vi "Write Rotronic.vi"(8 "error in":errorcluster, 10 "Rotronic":cluster{"RH":sgl, "T":sgl}, 11 "tCRD Data in":refnum<class "tCRD Data.lvclass">) -> (0 "error out":errorcluster, 3 "tCRD Data out":refnum<class "tCRD Data.lvclass">)   [LabVIEW 2015, in "tCRD Data.lvclass"]
uses:
  tCRD Data.lvclass
  tCRD Data.lvclass/tCRD Data.ctl
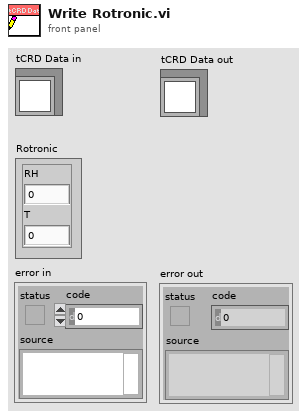
[diagram p1: front panel]
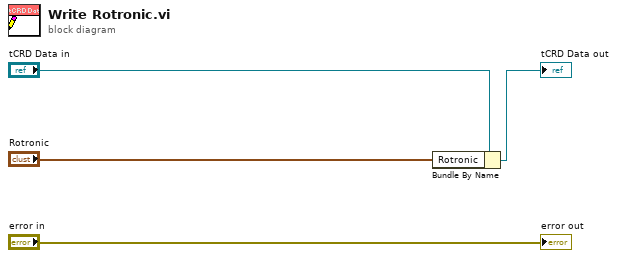
[diagram p0: block diagram]
diagram:
  n1 = Bundle By Name(cluster="tCRD Data in", "Rotronic"="Rotronic") -> (→"tCRD Data out":refnum<class "tCRD Data.lvclass">)
  "error out" <- "error in"
